vi "CPP_VeerSpectra.vi"() -> (5 "Plug in titles":string[](array[string]), 7 "Plug in values":string[](array[string]))   [LabVIEW 2021]
uses:
  Globals/Meas_global.vi
  Controls/Post_Process.ctl
  Acquisition/PWA/PWAtasksGLOBAL.vi
  Controls/Instrument_Array.ctl
  Controls/Graph_Type.ctl
panel:
  out "dF/ Hz":dbl
  in  "Inst Array":T1=enum."Analogue"
  in  "Show Smooth":bool=TRUE
  in  "Save Spectra?":bool
  in  "Desired number of samples per block":i32=32768
  in  "Calculate Spectra and Histogram?":bool=TRUE
  out "Spectra":cluster{dbl, dbl, "Spectrum output array":dbl[]}(graph)
  in  "Averaging samples":i32=1 min=1 max=1000
  in  "Spectra Index (from ALL channels)":i32
  out "Waveform Graph":dbl[][](graph)
  in  "Channels to Plot":i32[](array[ring])=[0, 1, 2, 3] items=["RV (Mic1)", "RV (Mic2)", "RV (Mic3)", "RV (Mic4)", "Save Nothing"]
  # "Run this VI to update the channel names"
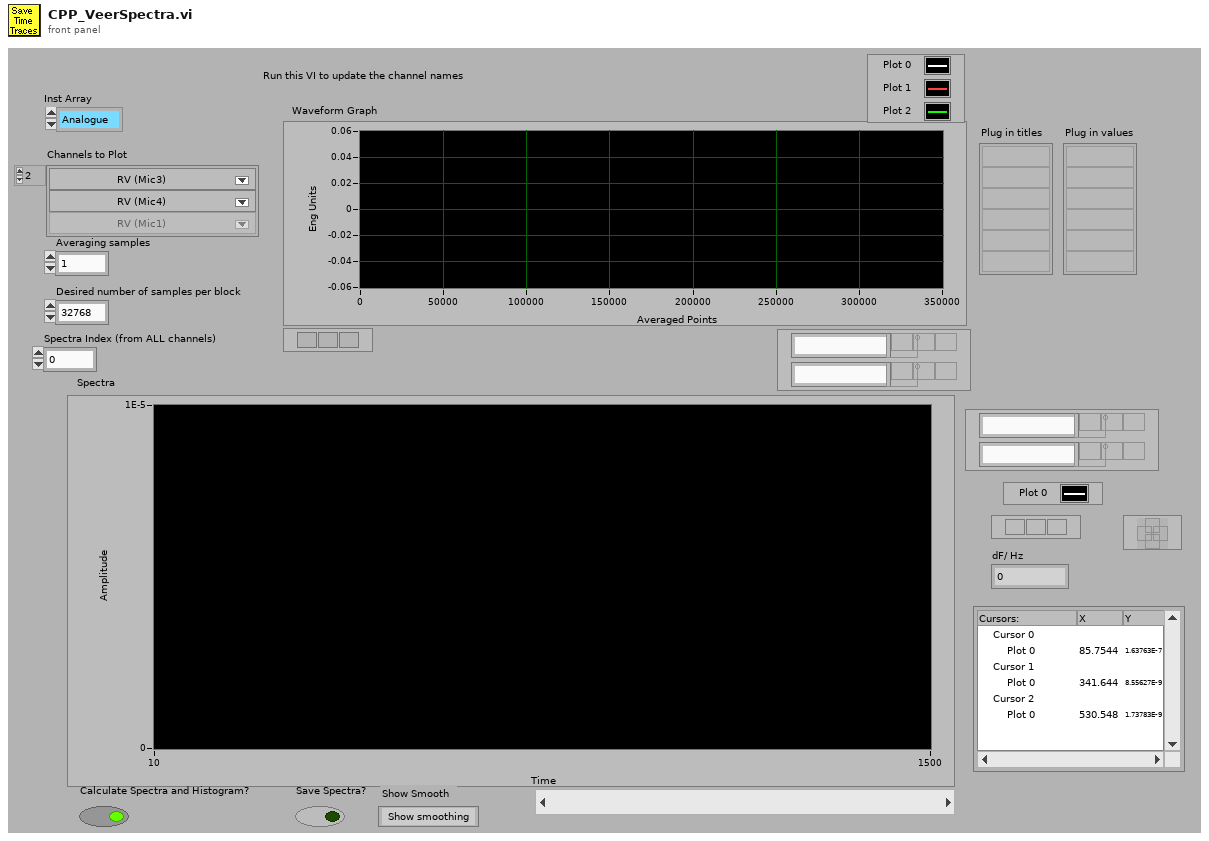
[diagram p1: front panel]
types:
  T1 = typedef "Instrument_Array.ctl" = enum16{"PWA", "LDA", "Analogue"}
  T2 = typedef "Analysis_info_cluster.ctl" = cluster{"Colour":u32, "Inst type":T3, "Inst name":string, "Symbol":string, "Code name":string, "Extra Info":string, "Inst Array":T1, "Extra Titles":string[], "Extra Values":string[], "U":dbl, "u^2":dbl, "u^3":dbl, "u^4":dbl, "Skew_u":dbl, "Kurt_u":dbl, "Sd Error in Mean":dbl, "% u'/U":dbl, "X":dbl, "Y":dbl, "Z":dbl, "Timescale integral Estimate":dbl, "Sd Error in Variance":dbl, "Calib File":path, "Calib Constants":dbl[], "Output Position":bool, "Stats":enum16{"None", "Basic", "Full"}, "Av Sampling Rate":dbl, "Av No of Samples":dbl, "Total Meas Time (s)":dbl, "ADAM Ch Name":string, "Max value":dbl, "Min value":dbl, "Req Sample Rate Hz":dbl, "Sync Delay Time (s)":dbl, "Ch No":i16, "Device":string, "Use Latest Calib":bool, "Port":string, "Metadata Ch Names":string[], "Metadata Ch Values":string[], "Label":string}
  T3 = typedef "Inst_type.ctl" = enum16{"Raw voltage", "Raw with zero offsetting", "Propeller anemometer", "Pressure Transducer", "Pitot-static tube", "Hot wire", "Cross wire 1", "Cross wire 2", "Generic Linear", "Generic Polynomial", "Generic BackPoly", "Fast FID", "Thermocouple", "Cold wire", "Pulsed Wire", "LDA Vel", "LDA Tran time", "LDA Arr time", "Microphone"}
  T4 = typedef "Post_Process.ctl" = enum16{"Take New Data", "Post Process Raw Data File"}
  T5 = typedef "Graph_Type.ctl" = enum16{"Show no graph", "Voltage trace", "Velocity trace", "Vel histogram", "Spectrum", "f.E(f) v Log f", "Auto-Corr"}
  T6 = cluster{"Plot 1":u16, "Plot 2":u16, "Save graph":u16, "Plot Type":T5}
  T7 = typedef "Time_Trace_Cluster.ctl" = cluster{"Weighting":dbl[], "Voltage":dbl[], "Eng Values":dbl[]}
  T8 = cluster{dbl, dbl, "Spectrum output array":dbl[]}[]
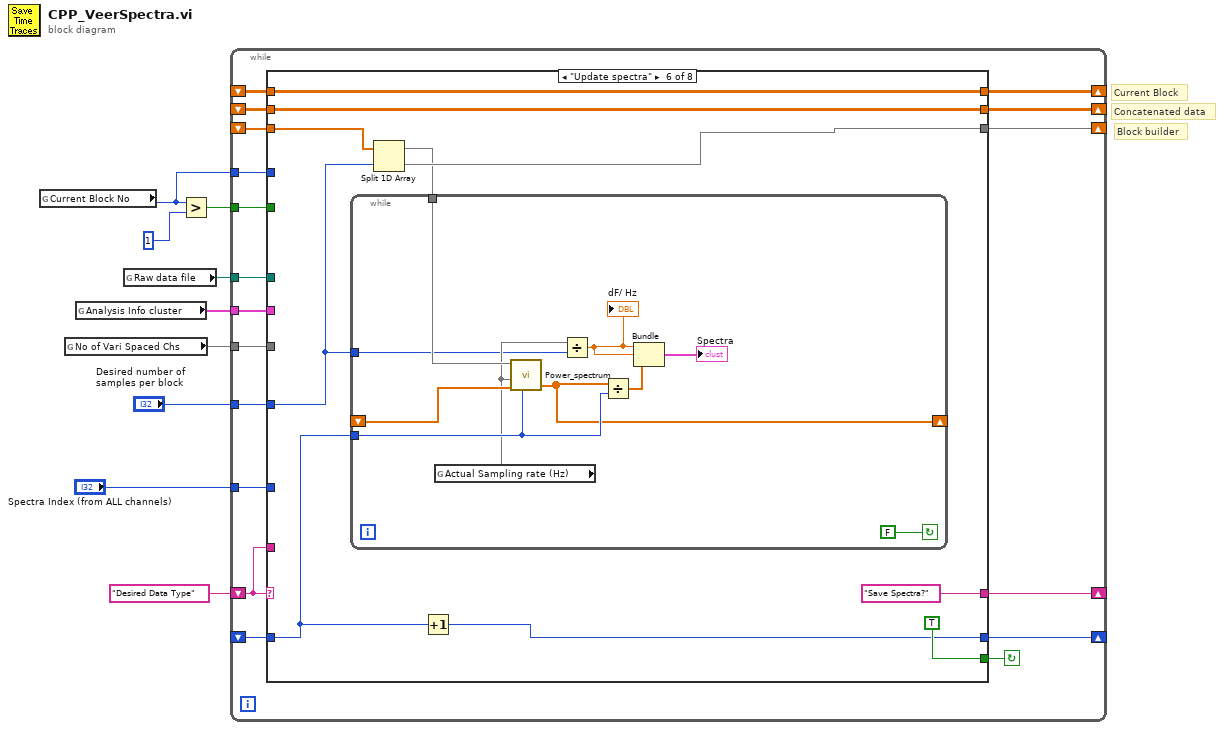
[diagram p0: block diagram]
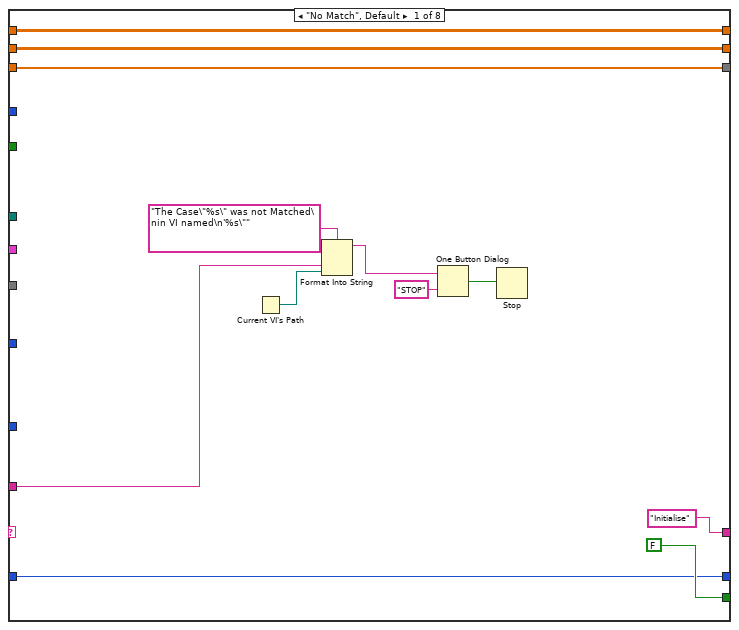
[diagram p2: hidden frame]
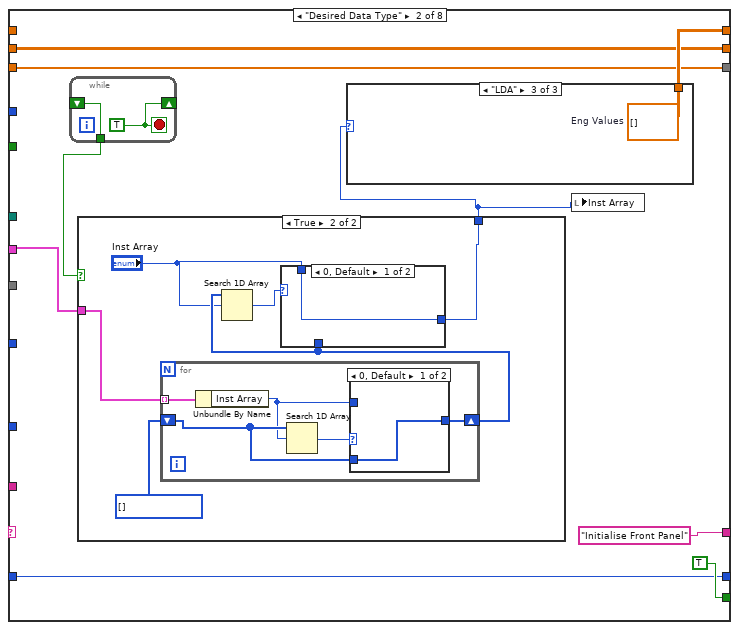
[diagram p3: hidden frame]
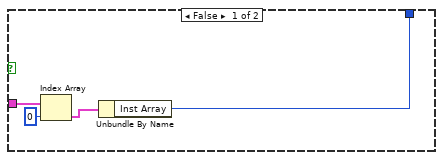
[diagram p4: hidden frame]
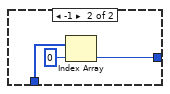
[diagram p5: hidden frame]
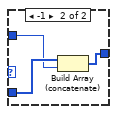
[diagram p6: hidden frame]
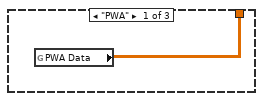
[diagram p7: hidden frame]
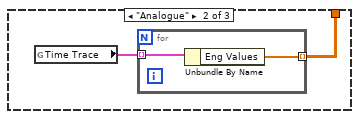
[diagram p8: hidden frame]
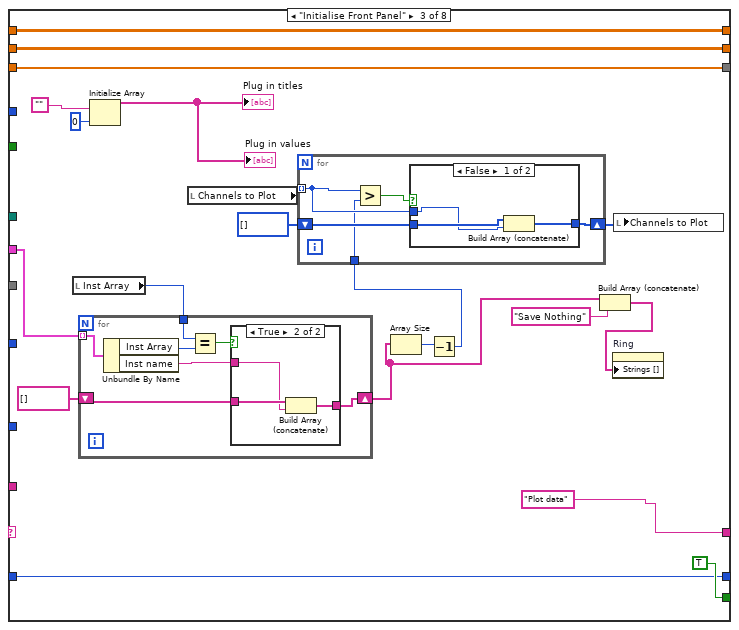
[diagram p9: hidden frame]
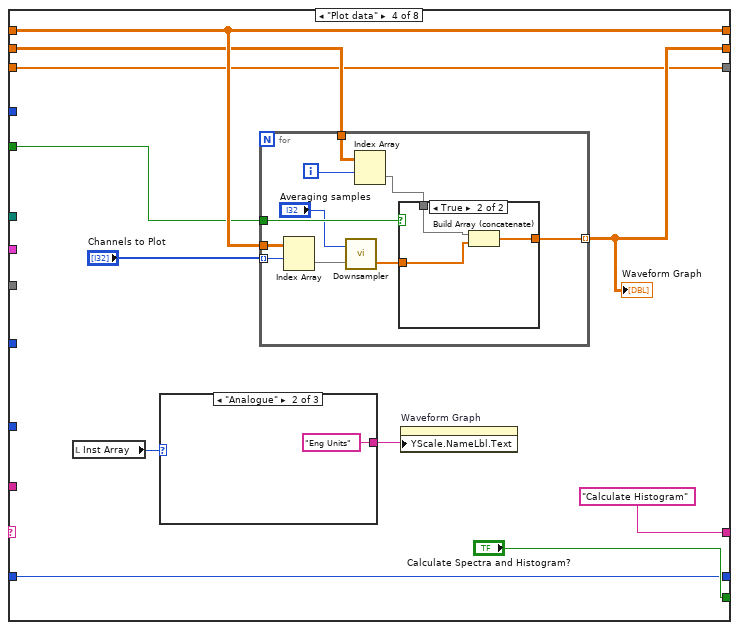
[diagram p12: hidden frame]
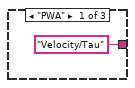
[diagram p13: hidden frame]
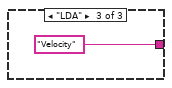
[diagram p14: hidden frame]
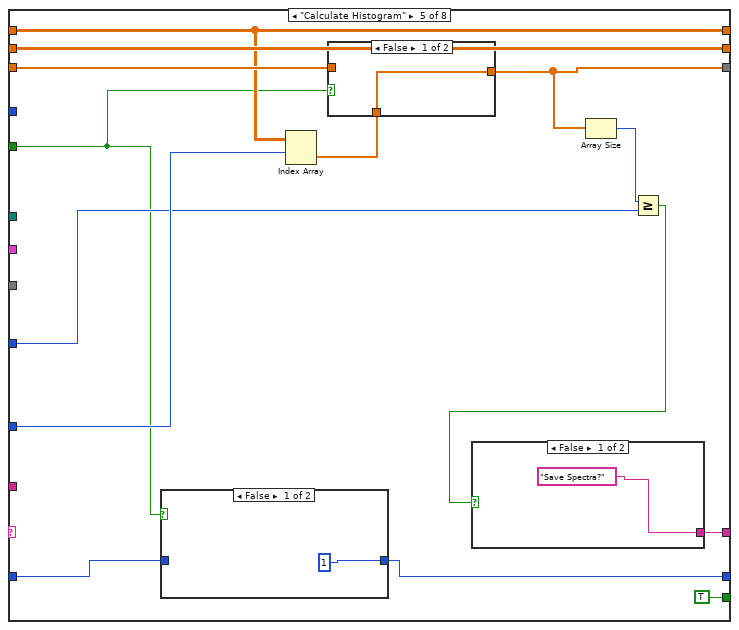
[diagram p16: hidden frame]
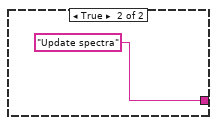
[diagram p18: hidden frame]
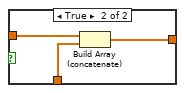
[diagram p19: hidden frame]
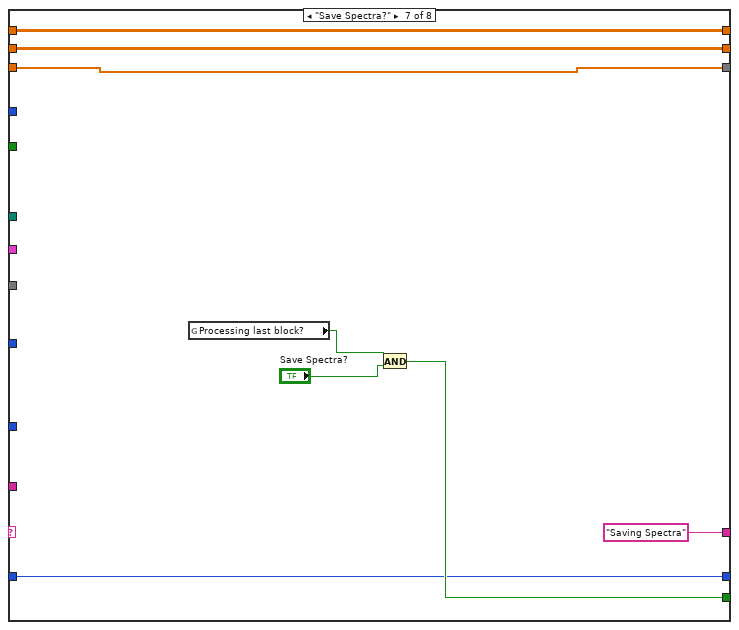
[diagram p20: hidden frame]
diagram:
  # "Block builder"
  # "Concatenated data"
  # "Current Block"
  n1 = global read "Meas_global.vi" "Current Block No"() -> (w6:i32)
  n2 = global read "Meas_global.vi" "No of Vari Spaced Chs"() -> (w4)
  n3 = global read "Meas_global.vi" "Analysis Info cluster"() -> (w5:T2[])
  n4 = global read "Meas_global.vi" "Raw data file"() -> (w8:path)
  n5 = Greater?(x=w6, y=1) -> (0:w3:bool)
  n6 = while {
    shift-left: "Desired Data Type" -> [w25]
    shift-right: [w26] -> _
    tunnel: w8 -> [w24]
    tunnel: w3 -> [w23]
    tunnel: w6 -> [w22]
    tunnel: w5 -> [w21]
    tunnel: w4 -> [w20]
    shift-right: [w19] -> _
    shift-left: _ -> [w18]
    shift-right: [w16] -> _
    shift-left: _ -> [w17]
    shift-right: [w14] -> _
    shift-left: _ -> [w15]
    tunnel: "Desired number of samples per block" -> [w13]
    tunnel: "Spectra Index (from ALL channels)" -> [w12]
    shift-right: [w11] -> _
    shift-left: _ -> [w10]
    stop <- w27 continue-if-true
    n7 = case shown="\"Update spectra\"" w25 {
      tunnel: [FALSE TRUE TRUE "Calculate Spectra and Histogram?" TRUE ("Calculate Spectra and Histogram?") TRUE ("Calculate Spectra and Histogram?") w191 FALSE ("Calculate Spectra and Histogram?")] -> w27
      tunnel: ["Initialise" "Initialise Front Panel" "Plot data" "Calculate Histogram" ("t") w151 "Save Spectra?" "Saving Spectra" w204] -> w26
      tunnel: w25 -> [w34 _ _ _ _ _ _ _]
      tunnel: w24 -> [_ _ _ _ _ _ _ _]
      tunnel: w23 -> [_ _ _ w128 w150 _ _ _]
      tunnel: w22 -> [_ _ _ _ _ _ _ _]
      tunnel: w21 -> [_ w41 w83 _ _ _ _ w202]
      tunnel: w20 -> [_ _ _ _ _ _ _ _]
      tunnel: [w31 w46 w89 w130 w159 w178 w196 w205] -> w19
      tunnel: w18 -> [w31 _ w89 w130 w159 w178 w196 w205]
      tunnel: w17 -> [w30 w45 w88 w129 w160 w179 w197 w206]
      tunnel: [w30 w45 w88 w126 w160 w179 w197 w206] -> w16
      tunnel: w15 -> [w29 w44 w85 w123 w161 w177 w194 w203]
      tunnel: [w29 w44 w85 w123 w157 w176 w194 w203] -> w14
      tunnel: w13 -> [_ _ _ _ w153 w172 _ w199]
      tunnel: w12 -> [_ _ _ _ w155 _ _ w201]
      tunnel: [w28 w43 w84 w122 w149 w170 w190 w198] -> w11
      tunnel: w10 -> [w28 w43 w84 w122 w148 w171 w190 w198]
      frame "No Match", Default {
        n8 = Current VI's Path() -> (path=w33:path)
        n9 = Format Into String(format string="The Case\"%s\" was not Matched\nin VI named\n'%s\"" ("Format String"), w34, w33) -> (resulting string=w37:string)  [unwired: 2 in, 1 out]
        n10 = One Button Dialog(message=w37, button name ("OK")="STOP") -> (true=w35:bool)
        n11 = Stop(stop? (T)=w35) -> ()
      }
      frame "Desired Data Type" {
        n12 = while {
          shift-right: [w73] -> _
          shift-left: _ -> [w72]
          tunnel: [w72] -> w42
          stop <- w73 stop-if-true
          w73 = TRUE
        }
        n13 = case shown="True" w42 {
          tunnel: w41 -> [w52 w58]
          tunnel: [w49 w54] -> w40
          frame False {
            n14 = Index Array(array=w52, index=0) -> (element=w50:T2)
            n15 = Unbundle By Name(w50) -> ("Inst Array"=w49:T1)
          }
          frame True {
            w57 = T1[] [] items=["PWA", "LDA", "Analogue"]
            n16 = for {
              tunnel: w58 -> [w67] mode=indexing
              shift-right: [w63] -> w55
              shift-left: w57 -> [w65]
              n17 = Unbundle By Name(w67) -> ("Inst Array"=w64:T1)
              n18 = Search 1D Array(1D array=w65, element=w64) -> (index of element=w66:i32)  [unwired: 1 out]
              n19 = case shown="0, Default" w66 {
                tunnel: w65 -> [w68 w71]
                tunnel: w64 -> [_ w70]
                tunnel: [w68 w69] -> w63
                frame 0, Default {
                }
                frame -1 {
                  n20 = Build Array (concatenate)(w71, w70) -> (w69:T1[])
                }
              }
            }
            n21 = Search 1D Array(1D array=w55, element="Inst Array") -> (index of element=w56:i32)  [unwired: 1 out]
            n22 = case shown="0, Default" w56 {
              tunnel: w55 -> [_ w61]
              tunnel: [w59 w60] -> w54
              tunnel: "Inst Array" -> [w59 _]
              frame 0, Default {
              }
              frame -1 {
                n23 = Index Array(array=w61, index=0) -> (element=w60:T1)
              }
            }
          }
        }
        n24 = case shown="\"LDA\"" w40 {
          tunnel: [w74 w75 w79] -> w46
          frame "PWA" {
            n25 = global read "PWAtasksGLOBAL.vi" "PWA Data"() -> (w74:dbl[][])
          }
          frame "Analogue" {
            n26 = global read "Meas_global.vi" "Time Trace"() -> (w76:T7[])
            n27 = for {
              tunnel: w76 -> [w78] mode=indexing
              tunnel: [w77] -> w75 mode=indexing
              n28 = Unbundle By Name(w78) -> ("Eng Values"=w77:dbl[])
            }
          }
          frame "LDA" {
            w79 = dbl[][] []  # Eng Values
          }
        }
        n29 = local write "Inst Array"(w40) -> ()
      }
      frame "Initialise Front Panel" {
        n30 = local read "Inst Array"() -> (w82:T1)
        n31 = for {
          tunnel: w82 -> [w105]
          tunnel: w83 -> [w104] mode=indexing
          shift-right: [w101] -> w81
          shift-left: string[] [] -> [w102]
          n32 = Unbundle By Name(w104) -> ("Inst Array"=w106:T1, "Inst name"=w100:string)
          n33 = Equal?(x=w105, y=w106) -> (x = y?=w103:bool)
          n34 = case shown="True" w103 {
            tunnel: w102 -> [w107 w110]
            tunnel: [w107 w109] -> w101
            tunnel: w100 -> [_ w108]
            frame False {
            }
            frame True {
              n35 = Build Array (concatenate)(w110, w108) -> (w109:string[])
            }
          }
        }
        n36 = Initialize Array("", 0) -> (→"Plug in values" →"Plug in titles":string[])
        n37 = local read "Channels to Plot"() -> (w96:i32[])
        n38 = Array Size(array=w81) -> (size(s)=w91:i32)
        n39 = Decrement(x=w91) -> (x-1=w90:i32)
        n40 = for {
          tunnel: w96 -> [w112] mode=indexing
          shift-right: [w113] -> w94
          shift-left: i32[] [] -> [w114]
          tunnel: w90 -> [w111]
          n41 = Greater?(x=w112, y=w111) -> (0:w115:bool)
          n42 = case shown="False" w115 {
            tunnel: w114 -> [w118 w119]
            tunnel: [w117 w119] -> w113
            tunnel: w112 -> [w116 _]
            frame False {
              n43 = Build Array (concatenate)(w118, w116) -> (w117:i32[])
            }
            frame True {
            }
          }
        }
        n44 = Build Array (concatenate)(w81, "Save Nothing") -> (w92:string[])
        n45 = property on="Ring" class="Ring (strict)"("Strings []"=w92) -> ()  [unwired: 2 in, 2 out]
        n46 = local write "Channels to Plot"(w94) -> ()
      }
      frame "Plot data" {
        n47 = local read "Inst Array"() -> (w121:T1)
        n48 = case shown="\"Analogue\"" w121 {
          tunnel: ["Velocity/Tau" "Eng Units" "Velocity"] -> w120
          frame "PWA" {
          }
          frame "Analogue" {
          }
          frame "LDA" {
          }
        }
        n49 = for {
          tunnel: w130 -> [w143]
          tunnel: "Channels to Plot" -> [w142] mode=indexing
          tunnel: w129 -> [w139]
          tunnel: [w140] -> w126 mode=indexing
          tunnel: w128 -> [w141]
          i -> [w138]
          n50 = Index Array(array=w143, index (row)=w142) -> (element=w136:dbl[])  [unwired: 1 in]
          n51 = call "Downsampler.vi"("Input Array"=w136, "Averaging samples"="Averaging samples") -> ("Downsampled Array"=w135:dbl[])  [unwired: 1 out]
          n52 = Index Array(array=w139, index (row)=w138) -> (element=w137:dbl[])  [unwired: 1 in]
          n53 = case shown="True" w141 {
            tunnel: w137 -> [_ w147]
            tunnel: w135 -> [w144 w146]
            tunnel: [w144 w145] -> w140
            frame False {
            }
            frame True {
              n54 = Build Array (concatenate)(w147, w146) -> (w145:dbl[])
            }
          }
        }
        "Waveform Graph" <- w126
        n55 = property on="Waveform Graph" class="WFGraph (strict)"("YScale.NameLbl.Text"=w120) -> ()  [unwired: 2 in, 2 out]
      }
      frame "Calculate Histogram" {
        n56 = case shown="False" w150 {
          tunnel: [1 w163] -> w149
          tunnel: w148 -> [_ w163]
          frame False {
          }
          frame True {
          }
        }
        n57 = Index Array(array=w159, index (row)=w155) -> (element=w158:dbl[])  [unwired: 1 in]
        n58 = case shown="False" w150 {
          tunnel: w161 -> [_ w169]
          tunnel: [w166 w168] -> w157
          tunnel: w158 -> [w166 w167]
          frame False {
          }
          frame True {
            n59 = Build Array (concatenate)(w169, w167) -> (w168:dbl[])
          }
        }
        n60 = Array Size(array=w157) -> (size(s)=w156:i32)
        n61 = Greater Or Equal?(x=w156, y=w153) -> (x >= y?=w152:bool)
        n62 = case shown="False" w152 {
          tunnel: ["Save Spectra?" ("f") "Update spectra"] -> w151
          frame False {
          }
          frame True {
          }
        }
      }
      frame "Update spectra" {
        n63 = Split 1D Array(array=w177, index=w172) -> (first subarray=w173:dbl[], second subarray=w176:dbl[])
        n64 = while {
          shift-left: _ -> [w187]
          shift-right: [w180] -> _
          tunnel: w173 -> [w188]
          tunnel: w171 -> [w186]
          tunnel: w172 -> [w184]
          stop <- FALSE continue-if-true
          n65 = global read "Meas_global.vi" "Actual Sampling rate (Hz)"() -> (w185)
          n66 = call "Power_spectrum.vi"("U"=w188, "Sampling frequency"=w185, "Spectrum input array"=w187, "Block No"=w186) -> ("Spectrum Accumulator array"=w180:dbl[])  [unwired: 1 in, 2 out]
          n67 = Divide(x=w185, y=w184) -> (x/y=w182:dbl)
          "dF/ Hz" <- w182
          n68 = Divide(x=w180, y=w186) -> (x/y=w181:dbl[])
          n69 = Bundle(w182, w182, w181) -> (→"Spectra":cluster{dbl, dbl, dbl[]})  [unwired: 1 out]
        }
        n70 = Increment(x=w171) -> (x+1=w170:i32)
      }
      frame "Save Spectra?" {
        n71 = global read "Meas_global.vi" "Processing last block?"() -> (w192:bool)
        n72 = And(x=w192, y="Save Spectra?") -> (x .and. y?=w191:bool)
      }
      frame "Saving Spectra" {
        n73 = stacked-sequence {
          seq-local: [w210 _ _ _] -> [_ _ w243 _]
          seq-local: [_ w230 _ _] -> [_ _ w242 _]
          tunnel: [_ _ "Save Spectra?" _] -> w204
          tunnel: w202 -> [_ _ w249 _]
          tunnel: w201 -> [_ _ w248 _]
          tunnel: w199 -> [w208 _ _ _]
          tunnel: w198 -> [_ w228 _ _]
          frame #0 {
            n74 = global read "Meas_global.vi" "Post Process"() -> (w212:T4)
            n75 = Equal?(x=w212, y=Post_Process."Take New Data" ("Post Process")) -> (x = y?=w213:bool)
            n76 = case shown="False" w213 {
              tunnel: [w221 w225] -> w214
              frame False {
                n77 = global read "Meas_global.vi" "Pre Setup String"() -> (w222:string)
                n78 = call "Get_value_from_string.vi"("Input string"=w222, "Variable name"="Seconds since 1/1/04") -> ("Value"=w221:dbl)  [unwired: 1 in, 1 out]
              }
              frame True {
                n79 = Get Date/Time In Seconds() -> (seconds since 1Jan1904=w224:timestamp)
                n80 = To Double Precision Float(number=w224) -> (double precision float=w225:dbl)
              }
            }
            n81 = To Unsigned Long Integer(number=w214) -> (unsigned 32bit integer=w218:u32)
            n82 = Get Date/Time String(date format (0)=enum16{"short", "long", "abbreviated"}."abbreviated", seconds (now)=w218) -> (date string=w216:string, time string=w217:string)  [unwired: 1 out]
            n83 = Number To Decimal String(number=w218) -> (decimal integer string=w219:string)  [unwired: 1 out]
            n84 = Number To Decimal String(number=w208) -> (decimal integer string=w207:string)  [unwired: 1 out]
            n85 = Build Array("Time of meas", w216, w217, w219, "Block Length" ("element"), w207) -> (w210:string[])
          }
          frame #1 {
            n86 = global read "Meas_global.vi" "Actual Sampling rate (Hz)"() -> (w231)
            n87 = Decrement(x=w228) -> (x-1=w227:i32)
            n88 = global read "Meas_global.vi" "Raw data file"() -> (w237:path)
            n89 = global read "Meas_global.vi" "Comments"() -> (w236:string)
            n90 = Number To Decimal String(number=w227) -> (decimal integer string=w226:string)  [unwired: 1 out]
            n91 = Number To Fractional String(number=w231, precision (6)=i16 2) -> (F-format string=w234:string)  [unwired: 2 out]
            n92 = call "Path_2_String.vi"("Real Path"=w237) -> ("Path String"=w238:string)
            n93 = Build Array("No of Blocks", w226, "Frequency (Hz)", w234, "Raw Data file", w238, w236) -> (w230:string[])
          }
          frame #2 {
            n94 = Index Array(array=w249, index=w248) -> (element=w247:T2)
            n95 = Unbundle By Name(w247) -> ("Inst name"=w246:string)
            n96 = Build Array (concatenate)(w243, w242) -> (w241:string[])
            n97 = Build Array(w246) -> (w245:string[])
            n98 = local read "Spectra"() -> (w252:cluster{dbl, dbl, "Spectrum output array":dbl[]})
            n99 = Build Array(w241) -> (w240:string[][])
            n100 = Build Array(w252) -> (w251:T8)
            n101 = call "Plot_to_file.vi"("Show Smooth"="Show Smooth", "Start trace No"=0, "Trace names"=w245, "Graph"=T6 {"Plot 1"=1, "Plot 2"=0, "Save graph"=1, "Plot Type"=enum."Spectrum"}, "Plot file label"=w240, "Plot data"=w251) -> ()  [unwired: 6 out]
          }
          frame #3 {
            n102 = local write "Show Smooth"(FALSE ("Show Smooth")) -> ()
          }
        }
      }
    }
  }
